vi "get shared variable name from url.vi"(8 "error in":errorcluster, 10 "string in":string) -> (0 "error out":errorcluster, 2 "Shared Variable":string)   [LabVIEW 2020]
uses:
  <vilib>/regexp/Match Regular Expression.xnode
panel:
  out "before match":string
  out "after match":string
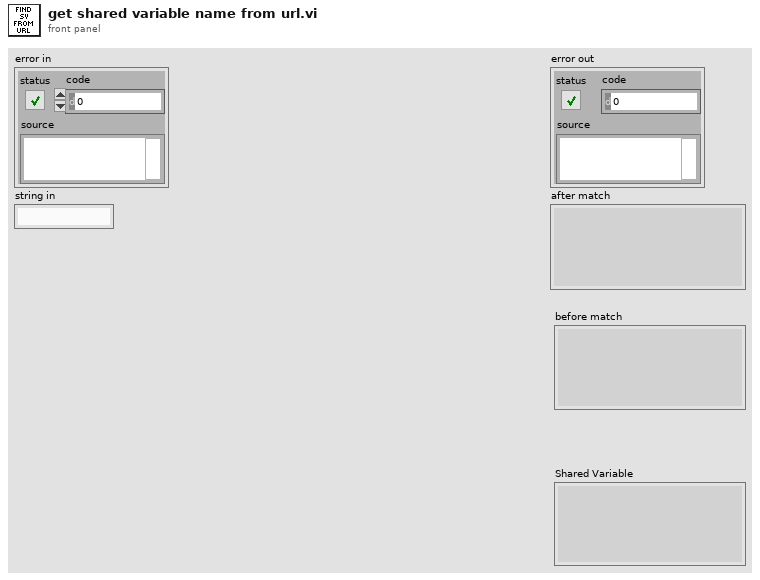
[diagram p1: front panel]
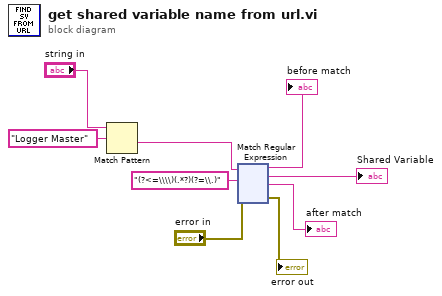
[diagram p0: block diagram]
diagram:
  n1 = Match Pattern(string="string in", regular expression="Logger Master") -> (after substring=w3:string)  [unwired: 1 in, 3 out]
  n2 = xnode "Match Regular Expression"("input string"=w3, "regular expression"="(?<=\\\\)(.*?)(?=\\.)", "error in"="error in") -> ("before match"=→"before match":string, "whole match"=→"Shared Variable":string, "after match"=→"after match":string, "error out"=→"error out":errorcluster)  [unwired: 3 in, 1 out]
